vi "tlc_File Module.vi"(7 "Command":T3, 8 "error in (no error)":errorcluster, 9 "Cue Array Input":T1[](array[typedef]) {"Channels"."Intensity" min=0.0 max=100.0 step=1.0 format="%#.0f"}, 10 "Path":path) -> (0 "error out":errorcluster, 1 "Cue Array Output":T1[](array[typedef]) {"Channels"."Intensity" min=0.0 max=100.0 step=1.0 format="%#.0f"})   [LabVIEW 2010]
uses:
  tlc_File_Command Control.ctl
  Controls/tlc_Cue_Information.ctl
  Controls/channel.ctl
panel:
  # "Local Data"
  # "Input Data"
  # "Output Data"
  # "No Local Data"
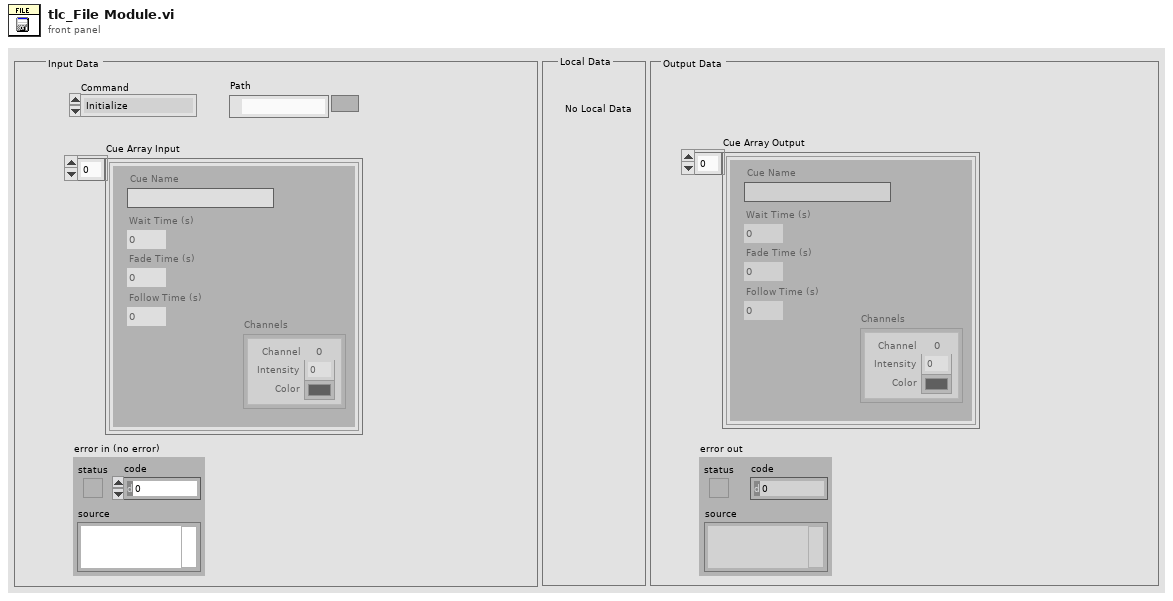
[diagram p1: front panel]
types:
  T1 = typedef "tlc_Cue_Information.ctl" = cluster{"Cue Name":string, "Wait Time (s)":u32, "Fade Time (s)":u32, "Follow Time (s)":u32, "Channels":T2[][]}
  T2 = typedef "channel.ctl" = cluster{"Intensity":dbl, " Color":u32, "Channel":i32}
  T3 = typedef "tlc_File_Command Control.ctl" = enum16{"Initialize", "Save Cues", "Load Cues", "Shutdown"}
  T4 = enum16{"open", "replace", "create", "open or create", "replace or create", "replace or create with confirmation"}
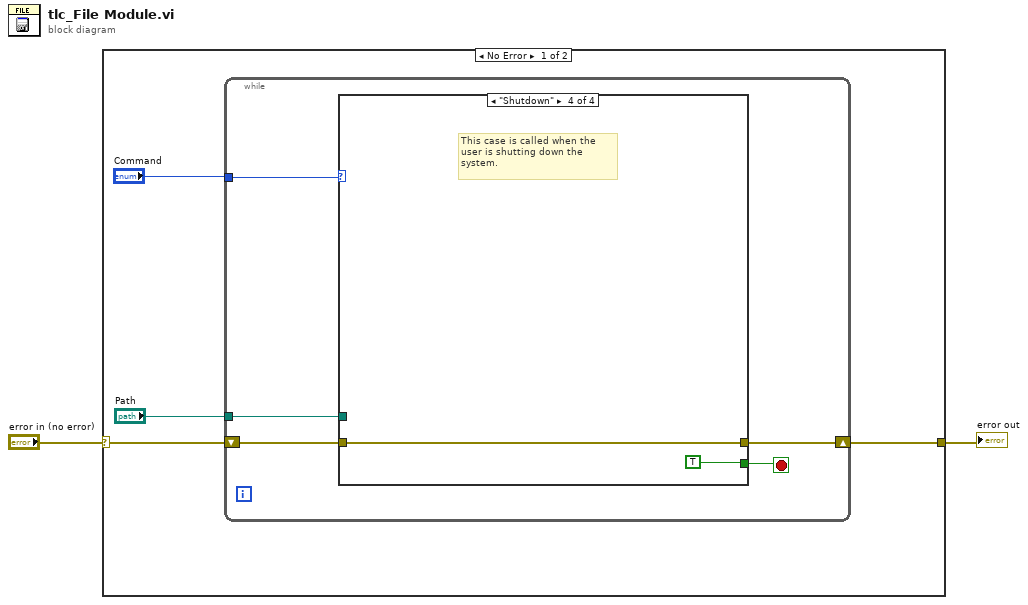
[diagram p0: block diagram]
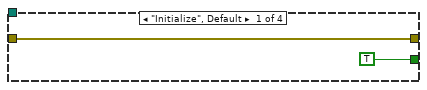
[diagram p2: hidden frame]
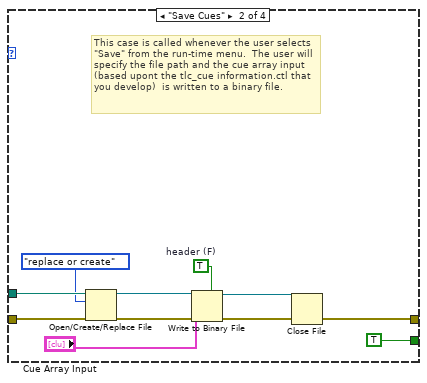
[diagram p3: hidden frame]
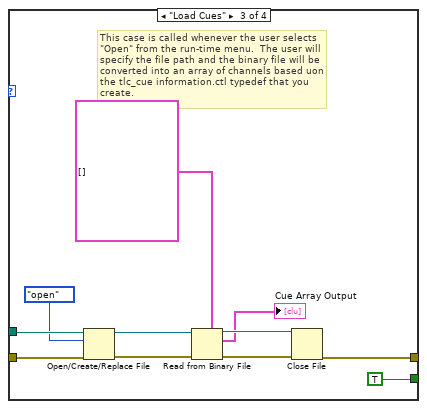
[diagram p4: hidden frame]
diagram:
  n1 = case shown="No Error" "error in (no error)" {
    selector: "error in (no error)" -> [w6 w38]
    tunnel: [w5 w38] -> w1
    frame No Error {
      n2 = while {
        shift-right: [w9] -> w5
        shift-left: w6 -> [w10]
        tunnel: "Path" -> [w8]
        tunnel: "Command" -> [w7]
        stop <- w11 stop-if-true
        n3 = case shown="\"Shutdown\"" w7 {
          tunnel: [TRUE TRUE TRUE TRUE] -> w11
          tunnel: w10 -> [w12 w17 w29 w37]
          tunnel: [w12 w16 w28 w37] -> w9
          tunnel: w8 -> [_ w23 w34 _]
          frame "Initialize", Default {
          }
          frame "Save Cues" {
            w18 = TRUE  # header (F)
            # "This case is called whenever the user selects \"Save\" from the run-time menu.  The user will specify the file path and the cue array input (based upont the tlc_cue information.ctl that you develop)  is written to a binary file."
            n4 = Open/Create/Replace File(file path (use dialog)=w23, error in=w17, operation (0:open)=T4."replace or create") -> (refnum out=w22:refnum<file>, error out=w19:errorcluster)  [unwired: 3 in, 1 out]
            n5 = Write to Binary File(file (use dialog)=w22, data="Cue Array Input", error in=w19, 5:w18) -> (refnum out=w21:refnum<file>, error out=w20:errorcluster)  [unwired: 2 in, 1 out]
            n6 = Close File(refnum=w21, error in=w20) -> (error out=w16:errorcluster)  [unwired: 1 out]
          }
          frame "Load Cues" {
            # "This case is called whenever the user selects \"Open\" from the run-time menu.  The user will specify the file path and the binary file will be converted into an array of channels based uon the tlc_cue information.ctl typedef that you create."
            n7 = Open/Create/Replace File(file path (use dialog)=w34, error in=w29, operation (0:open)=T4."open") -> (refnum out=w33:refnum<file>, error out=w31:errorcluster)  [unwired: 3 in, 1 out]
            n8 = Read from Binary File(5:T1[] [], 8:w31, 11:w33) -> (0:w30:errorcluster, 2:→"Cue Array Output":T1[], 3:w32:refnum<file>)  [unwired: 3 in, 1 out]
            n9 = Close File(refnum=w32, error in=w30) -> (error out=w28:errorcluster)  [unwired: 1 out]
          }
          frame "Shutdown" {
            # "This case is called when the user is shutting down the system."
          }
        }
      }
    }
    frame Error {
    }
  }
  "error out" <- w1
